vi "czyWWezu.vi"(10 "kordyPunktu":cluster{dbl, dbl}, 11 "kordyCiala":cluster{"Width":dbl, "Height":dbl}[](array[cluster])) -> (3 "czyNaszedl?":bool)   [LabVIEW 2020]
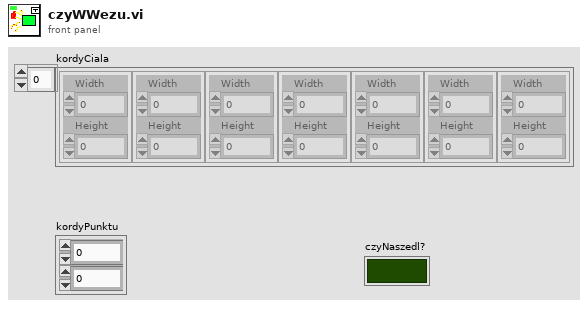
[diagram p1: front panel]
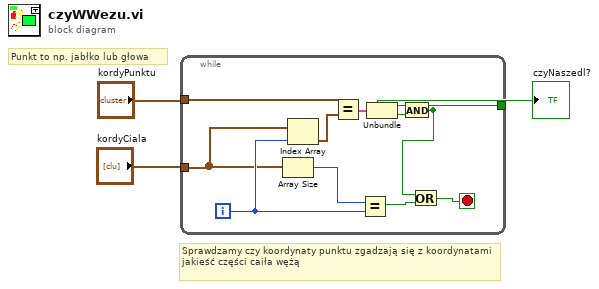
[diagram p0: block diagram]
diagram:
  # "Sprawdzamy czy koordynaty punktu zgadzają się z koordynatami jakieść części caiła wężą"
  # "Punkt to np. jabłko lub głowa"
  n1 = while {
    tunnel: "kordyPunktu" -> [w8]
    tunnel: "kordyCiala" -> [w10]
    tunnel: [w4] -> w3
    i -> [w11]
    stop <- w14 stop-if-true
    n2 = Array Size(array=w10) -> (size(s)=w13:i32)
    n3 = Index Array(array=w10, index=w11) -> (element=w9:cluster{"Width":dbl, "Height":dbl})
    n4 = Equal?(x=w8, y=w9) -> (x = y?=w7:cluster{bool, bool})
    n5 = Equal?(x=w13, y=w11) -> (x = y?=w12:bool)
    n6 = Unbundle(w7) -> (w6:bool, w5:bool)
    n7 = And(x=w6, y=w5) -> (x .and. y?=w4:bool)
    n8 = Or(x=w4, y=w12) -> (x .or. y?=w14:bool)
  }
  "czyNaszedl?" <- w3
